vi "Servicio Estatus Tabla.vi"(8 "error in":errorcluster, 10 "Servicio Estatus":string[][](array[string])) -> (0 "error out":errorcluster)   [LabVIEW 2020, in "Contabilidad.lvlib"]
doc: "_____\nCreated using DQMH Event Scripter 6.0.0.122."
uses:
  Contabilidad.lvlib
  Servicio Estatus Tabla Argument--cluster.ctl
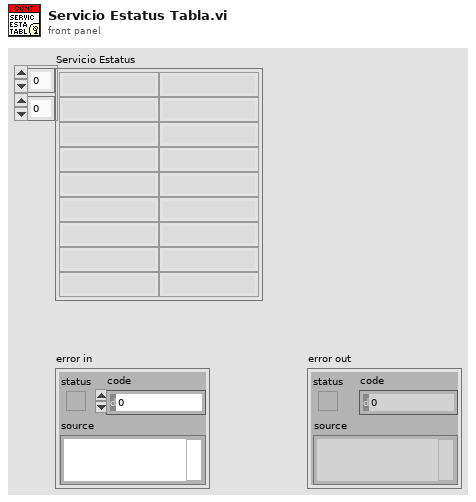
[diagram p1: front panel]
types:
  T1 = typedef "Contabilidad.lvlib/Servicio Estatus Tabla Argument--cluster.ctl" = cluster{"Servicio Estatus":string[][]}
  T2 = typedef "Contabilidad.lvlib/Broadcast Events--cluster.ctl" = cluster{"Module Did Init":refnum<user-event>, "Status Updated":refnum<user-event>, "Error Reported":refnum<user-event>, "Module Did Stop":refnum<user-event>, "Update Module Execution Status":refnum<user-event>, "Servicio Estatus Tabla":refnum<user-event>}
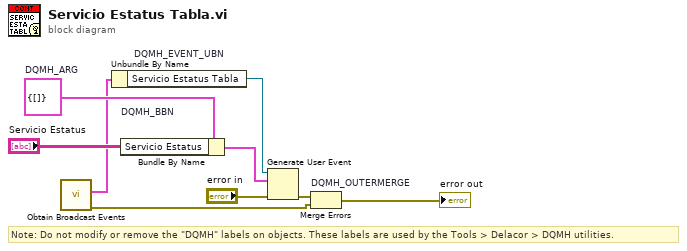
[diagram p0: block diagram]
diagram:
  w4 = T1 {"Servicio Estatus"=[]}  # DQMH_ARG
  # "Note: Do not modify or remove the \"DQMH\" labels on objects. These labels are used by the Tools > Delacor > DQMH utilities."
  n1 = call "Obtain Broadcast Events.vi"() -> ("error out"=w2:errorcluster, "Contabilidad Broadcast Events"=w1:T2)  [unwired: 10 in]
  n2 = Unbundle By Name "DQMH_EVENT_UBN"(w1) -> ("Servicio Estatus Tabla"=w6:refnum<user-event>)
  n3 = Bundle By Name "DQMH_BBN"(cluster=w4, "Servicio Estatus"="Servicio Estatus") -> (w7:T1)
  n4 = Generate User Event(user event=w6, event data cluster=w7, error in="error in") -> (error out=w5:errorcluster)  [unwired: 1 in, 1 out]
  n5 = Merge Errors "DQMH_OUTERMERGE"(w5, w2) -> (→"error out":errorcluster)
